vi "Result.Attribute, Compare Value to Limits.vi"(8 "UL":string, 9 "LL":string, 10 "Value":string, 11 "LimType":T2) -> (1 "Desc":string, 3 "Status":T1=3 items=["LOG", "PASS", "FAIL", "ERROR"])   [LabVIEW 2018]
uses:
  Result.Limit Type.ctl
  Result.Measurement and Attribute Item Status.ctl
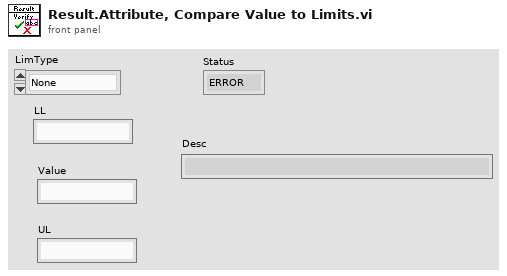
[diagram p1: front panel]
types:
  T1 = typedef "Result.Measurement and Attribute Item Status.ctl" = i32
  T2 = typedef "Result.Limit Type.ctl" = enum16{"None", "EQ", "NE", "GT", "LT", "GE", "LE", "GTLT", "GELE", "GELT", "GTLE", "LTGT", "LEGE", "LEGT", "LTGE", "Contains", "NotContains"}
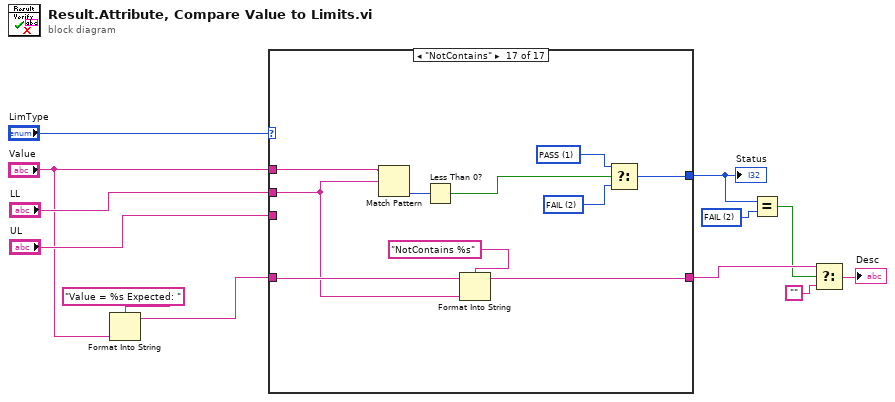
[diagram p0: block diagram]
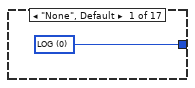
[diagram p2: hidden frame]
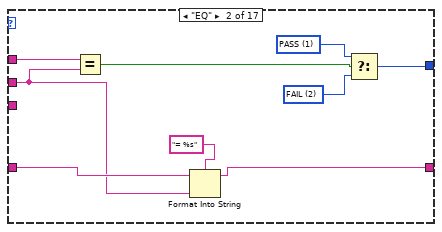
[diagram p3: hidden frame]
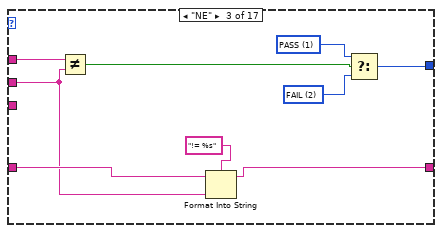
[diagram p4: hidden frame]
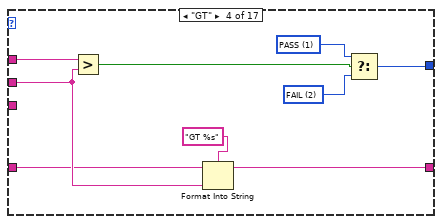
[diagram p5: hidden frame]
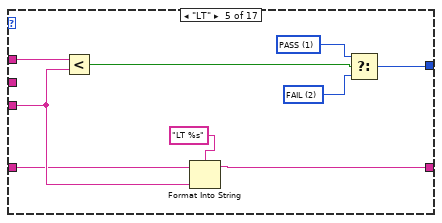
[diagram p6: hidden frame]
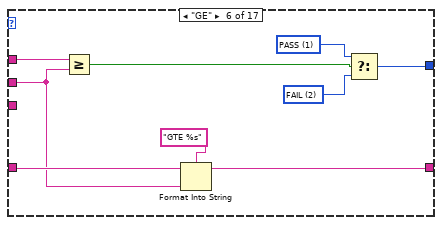
[diagram p7: hidden frame]
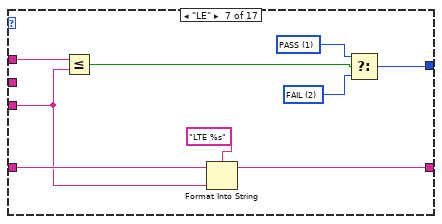
[diagram p8: hidden frame]
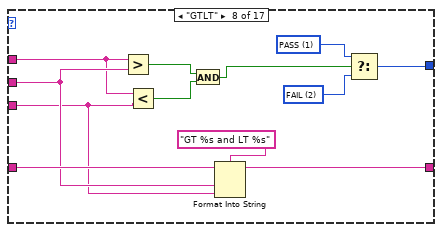
[diagram p9: hidden frame]
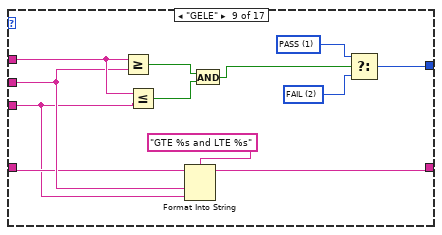
[diagram p10: hidden frame]
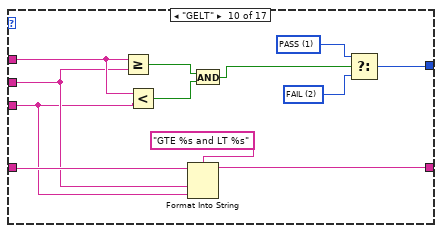
[diagram p11: hidden frame]
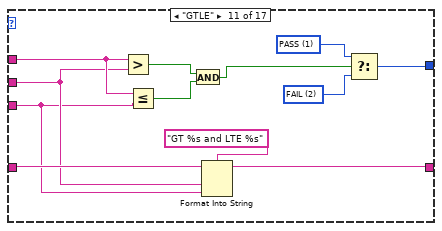
[diagram p12: hidden frame]
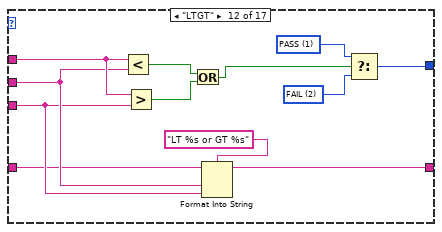
[diagram p13: hidden frame]
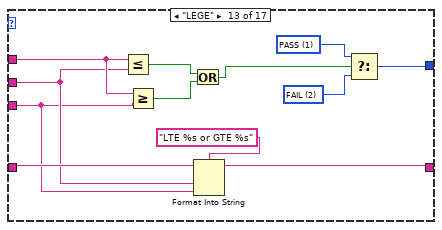
[diagram p14: hidden frame]
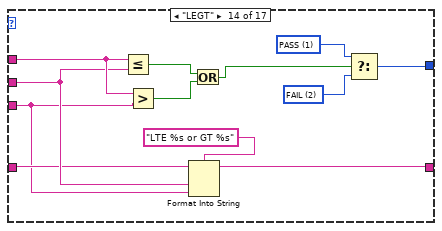
[diagram p15: hidden frame]
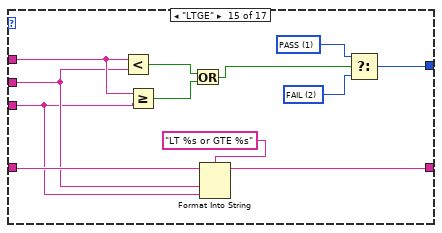
[diagram p16: hidden frame]
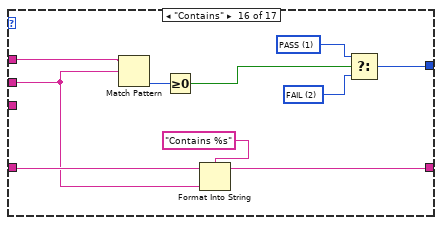
[diagram p17: hidden frame]
diagram:
  w5 = T1 2 items=["LOG", "PASS", "FAIL", "ERROR"] ("Status")
  n1 = Format Into String(format string="Value = %s Expected: ", "Value") -> (resulting string=w9:string)  [unwired: 2 in, 1 out]
  n2 = case shown="\"NotContains\"" "LimType" {
    tunnel: "Value" -> [_ w17 w31 w40 w49 w54 w63 w69 w85 w97 w112 w124 w136 w148 w160 w167 w177]
    tunnel: "LL" -> [_ w14 w24 w34 _ w50 _ w70 w83 w93 w105 w119 w129 w142 w153 w166 w176]
    tunnel: "UL" -> [_ _ _ _ w42 _ w60 w68 w81 w92 w104 w118 w128 w140 w152 _ _]
    tunnel: [w13 w22 w30 w39 w48 w58 w67 w79 w91 w103 w115 w127 w139 w151 w163 w173 w183] -> w6
    tunnel: [_ w15 w23 w33 w43 w51 w59 w72 w80 w95 w106 w116 w130 w143 w154 w168 w178] -> w3
    tunnel: w9 -> [_ w16 w25 w32 w41 w52 w61 w71 w82 w94 w107 w117 w131 w141 w155 w169 w179]
    frame "None", Default {
      w13 = T1 0 items=["LOG", "PASS", "FAIL", "ERROR"] ("Status")
    }
    frame "EQ" {
      w20 = T1 2 items=["LOG", "PASS", "FAIL", "ERROR"] ("Status")
      w21 = T1 1 items=["LOG", "PASS", "FAIL", "ERROR"] ("Status")
      n3 = Equal?(x=w17, y=w14) -> (x = y?=w19:bool)
      n4 = Format Into String(format string="= %s", initial string=w16, w14) -> (resulting string=w15:string)  [unwired: 1 in, 1 out]
      n5 = Select(t=w21, s=w19, f=w20) -> (s? t:f=w22:T1)
    }
    frame "NE" {
      w28 = T1 2 items=["LOG", "PASS", "FAIL", "ERROR"] ("Status")
      w29 = T1 1 items=["LOG", "PASS", "FAIL", "ERROR"] ("Status")
      n6 = Not Equal?(x=w31, y=w24) -> (x != y?=w27:bool)
      n7 = Format Into String(format string="!= %s", initial string=w25, w24) -> (resulting string=w23:string)  [unwired: 1 in, 1 out]
      n8 = Select(t=w29, s=w27, f=w28) -> (s? t:f=w30:T1)
    }
    frame "GT" {
      w37 = T1 2 items=["LOG", "PASS", "FAIL", "ERROR"] ("Status")
      w38 = T1 1 items=["LOG", "PASS", "FAIL", "ERROR"] ("Status")
      n9 = Greater?(x=w40, y=w34) -> (0:w36:bool)
      n10 = Format Into String(format string="GT %s", initial string=w32, w34) -> (resulting string=w33:string)  [unwired: 1 in, 1 out]
      n11 = Select(t=w38, s=w36, f=w37) -> (s? t:f=w39:T1)
    }
    frame "LT" {
      w46 = T1 2 items=["LOG", "PASS", "FAIL", "ERROR"] ("Status")
      w47 = T1 1 items=["LOG", "PASS", "FAIL", "ERROR"] ("Status")
      n12 = Less?(x=w49, y=w42) -> (x < y?=w45:bool)
      n13 = Format Into String(format string="LT %s", initial string=w41, w42) -> (resulting string=w43:string)  [unwired: 1 in, 1 out]
      n14 = Select(t=w47, s=w45, f=w46) -> (s? t:f=w48:T1)
    }
    frame "GE" {
      w56 = T1 2 items=["LOG", "PASS", "FAIL", "ERROR"] ("Status")
      w57 = T1 1 items=["LOG", "PASS", "FAIL", "ERROR"] ("Status")
      n15 = Greater Or Equal?(x=w54, y=w50) -> (x >= y?=w55:bool)
      n16 = Format Into String(format string="GTE %s", initial string=w52, w50) -> (resulting string=w51:string)  [unwired: 1 in, 1 out]
      n17 = Select(t=w57, s=w55, f=w56) -> (s? t:f=w58:T1)
    }
    frame "LE" {
      w65 = T1 2 items=["LOG", "PASS", "FAIL", "ERROR"] ("Status")
      w66 = T1 1 items=["LOG", "PASS", "FAIL", "ERROR"] ("Status")
      n18 = Less Or Equal?(x=w63, y=w60) -> (x <= y?=w64:bool)
      n19 = Format Into String(format string="LTE %s", initial string=w61, w60) -> (resulting string=w59:string)  [unwired: 1 in, 1 out]
      n20 = Select(t=w66, s=w64, f=w65) -> (s? t:f=w67:T1)
    }
    frame "GTLT" {
      w77 = T1 2 items=["LOG", "PASS", "FAIL", "ERROR"] ("Status")
      w78 = T1 1 items=["LOG", "PASS", "FAIL", "ERROR"] ("Status")
      n21 = Greater?(x=w69, y=w70) -> (0:w76:bool)
      n22 = Less?(x=w69, y=w68) -> (x < y?=w75:bool)
      n23 = And(x=w76, y=w75) -> (x .and. y?=w74:bool)
      n24 = Format Into String(format string="GT %s and LT %s", initial string=w71, w70, w68) -> (resulting string=w72:string)  [unwired: 1 in, 1 out]
      n25 = Select(t=w78, s=w74, f=w77) -> (s? t:f=w79:T1)
    }
    frame "GELE" {
      w89 = T1 2 items=["LOG", "PASS", "FAIL", "ERROR"] ("Status")
      w90 = T1 1 items=["LOG", "PASS", "FAIL", "ERROR"] ("Status")
      n26 = Greater Or Equal?(x=w85, y=w83) -> (x >= y?=w88:bool)
      n27 = Less Or Equal?(x=w85, y=w81) -> (x <= y?=w87:bool)
      n28 = Format Into String(format string="GTE %s and LTE %s", initial string=w82, w83, w81) -> (resulting string=w80:string)  [unwired: 1 in, 1 out]
      n29 = And(x=w88, y=w87) -> (x .and. y?=w86:bool)
      n30 = Select(t=w90, s=w86, f=w89) -> (s? t:f=w91:T1)
    }
    frame "GELT" {
      w101 = T1 2 items=["LOG", "PASS", "FAIL", "ERROR"] ("Status")
      w102 = T1 1 items=["LOG", "PASS", "FAIL", "ERROR"] ("Status")
      n31 = Greater Or Equal?(x=w97, y=w93) -> (x >= y?=w100:bool)
      n32 = Less?(x=w97, y=w92) -> (x < y?=w99:bool)
      n33 = Format Into String(format string="GTE %s and LT %s", initial string=w94, w93, w92) -> (resulting string=w95:string)  [unwired: 1 in, 1 out]
      n34 = And(x=w100, y=w99) -> (x .and. y?=w98:bool)
      n35 = Select(t=w102, s=w98, f=w101) -> (s? t:f=w103:T1)
    }
    frame "GTLE" {
      w113 = T1 2 items=["LOG", "PASS", "FAIL", "ERROR"] ("Status")
      w114 = T1 1 items=["LOG", "PASS", "FAIL", "ERROR"] ("Status")
      n36 = Greater?(x=w112, y=w105) -> (0:w111:bool)
      n37 = Less Or Equal?(x=w112, y=w104) -> (x <= y?=w110:bool)
      n38 = And(x=w111, y=w110) -> (x .and. y?=w109:bool)
      n39 = Format Into String(format string="GT %s and LTE %s", initial string=w107, w105, w104) -> (resulting string=w106:string)  [unwired: 1 in, 1 out]
      n40 = Select(t=w114, s=w109, f=w113) -> (s? t:f=w115:T1)
    }
    frame "LTGT" {
      w125 = T1 2 items=["LOG", "PASS", "FAIL", "ERROR"] ("Status")
      w126 = T1 1 items=["LOG", "PASS", "FAIL", "ERROR"] ("Status")
      n41 = Less?(x=w124, y=w119) -> (x < y?=w123:bool)
      n42 = Greater?(x=w124, y=w118) -> (0:w122:bool)
      n43 = Or(x=w123, y=w122) -> (x .or. y?=w121:bool)
      n44 = Format Into String(format string="LT %s or GT %s", initial string=w117, w119, w118) -> (resulting string=w116:string)  [unwired: 1 in, 1 out]
      n45 = Select(t=w126, s=w121, f=w125) -> (s? t:f=w127:T1)
    }
    frame "LEGE" {
      w137 = T1 2 items=["LOG", "PASS", "FAIL", "ERROR"] ("Status")
      w138 = T1 1 items=["LOG", "PASS", "FAIL", "ERROR"] ("Status")
      n46 = Less Or Equal?(x=w136, y=w129) -> (x <= y?=w135:bool)
      n47 = Greater Or Equal?(x=w136, y=w128) -> (x >= y?=w134:bool)
      n48 = Or(x=w135, y=w134) -> (x .or. y?=w133:bool)
      n49 = Format Into String(format string="LTE %s or GTE %s", initial string=w131, w129, w128) -> (resulting string=w130:string)  [unwired: 1 in, 1 out]
      n50 = Select(t=w138, s=w133, f=w137) -> (s? t:f=w139:T1)
    }
    frame "LEGT" {
      w149 = T1 2 items=["LOG", "PASS", "FAIL", "ERROR"] ("Status")
      w150 = T1 1 items=["LOG", "PASS", "FAIL", "ERROR"] ("Status")
      n51 = Less Or Equal?(x=w148, y=w142) -> (x <= y?=w147:bool)
      n52 = Greater?(x=w148, y=w140) -> (0:w146:bool)
      n53 = Format Into String(format string="LTE %s or GT %s", initial string=w141, w142, w140) -> (resulting string=w143:string)  [unwired: 1 in, 1 out]
      n54 = Or(x=w147, y=w146) -> (x .or. y?=w145:bool)
      n55 = Select(t=w150, s=w145, f=w149) -> (s? t:f=w151:T1)
    }
    frame "LTGE" {
      w161 = T1 2 items=["LOG", "PASS", "FAIL", "ERROR"] ("Status")
      w162 = T1 1 items=["LOG", "PASS", "FAIL", "ERROR"] ("Status")
      n56 = Less?(x=w160, y=w153) -> (x < y?=w159:bool)
      n57 = Greater Or Equal?(x=w160, y=w152) -> (x >= y?=w158:bool)
      n58 = Or(x=w159, y=w158) -> (x .or. y?=w157:bool)
      n59 = Format Into String(format string="LT %s or GTE %s", initial string=w155, w153, w152) -> (resulting string=w154:string)  [unwired: 1 in, 1 out]
      n60 = Select(t=w162, s=w157, f=w161) -> (s? t:f=w163:T1)
    }
    frame "Contains" {
      w171 = T1 2 items=["LOG", "PASS", "FAIL", "ERROR"] ("Status")
      w172 = T1 1 items=["LOG", "PASS", "FAIL", "ERROR"] ("Status")
      n61 = Match Pattern(string=w167, regular expression=w166) -> (offset past match=w165:i32)  [unwired: 1 in, 3 out]
      n62 = Greater Or Equal To 0?(x=w165) -> (x >= 0?=w164:bool)
      n63 = Format Into String(format string="Contains %s", initial string=w169, w166) -> (resulting string=w168:string)  [unwired: 1 in, 1 out]
      n64 = Select(t=w172, s=w164, f=w171) -> (s? t:f=w173:T1)
    }
    frame "NotContains" {
      w181 = T1 2 items=["LOG", "PASS", "FAIL", "ERROR"] ("Status")
      w182 = T1 1 items=["LOG", "PASS", "FAIL", "ERROR"] ("Status")
      n65 = Match Pattern(string=w177, regular expression=w176) -> (offset past match=w175:i32)  [unwired: 1 in, 3 out]
      n66 = Less Than 0?(x=w175) -> (x < 0?=w174:bool)
      n67 = Format Into String(format string="NotContains %s", initial string=w179, w176) -> (resulting string=w178:string)  [unwired: 1 in, 1 out]
      n68 = Select(t=w182, s=w174, f=w181) -> (s? t:f=w183:T1)
    }
  }
  "Status" <- w6
  n69 = Equal?(x=w6, y=w5) -> (x = y?=w2:bool)
  n70 = Select(t=w3, s=w2, f="") -> (s? t:f=→"Desc":string)
